vi "Save Archiving Parameters.vi"(5 "section":string, 7 "config ref in":T1, 8 "error in (no error)":errorcluster, 9 "2 LBCB Archiving Mode":bool, 10 "Log File Size (MBytes)":i64, 11 "Logging Directory":path) -> (0 "error out":errorcluster, 1 "config ref out":T1)   [LabVIEW 2013]
uses:
  <vilib>/Utility/config.llb/Config Data RefNum.ctl
  <vilib>/Utility/config.llb/Write Key (Path).vi
  <vilib>/Utility/config.llb/Write Key (Double).vi
  <vilib>/Utility/config.llb/Write Key (Boolean).vi
  <vilib>/Utility/config.llb/NI_LVConfig.lvlib
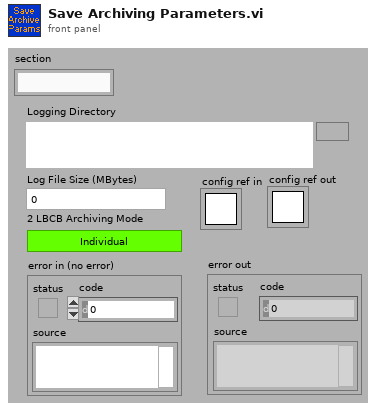
[diagram p1: front panel]
types:
  T1 = typedef "NI_LVConfig.lvlib/Config Data RefNum.ctl" = refnum<k1>
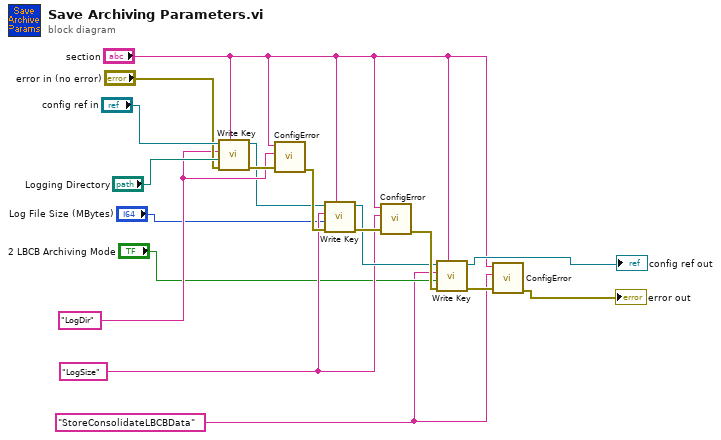
[diagram p0: block diagram]
diagram:
  w1 = "StoreConsolidateLBCBData" ("key")
  w4 = "LogSize" ("key")
  w14 = "LogDir" ("key")
  n1 = call-poly <vilib>:"Write Key.vi"("section"="section", "error in (no error)"="error in (no error)", "value"="Logging Directory", "key"=w14, "refnum"="config ref in") -> ("error out"=w15:errorcluster, "refnum out"=w8:T1)  [unwired: 4 in, 1 out]
  n2 = call "ConfigError.vi"("error in (no error)"=w15, "Key"=w14, "Section"="section") -> ("error out"=w11:errorcluster)  [unwired: 8 in]
  n3 = call-poly <vilib>:"Write Key.vi"("section"="section", "error in (no error)"=w11, "value"="Log File Size (MBytes)", "key"=w4, "refnum"=w8) -> ("error out"=w13:errorcluster, "refnum out"=w7:T1)  [unwired: 4 in, 1 out]
  n4 = call "ConfigError.vi"("error in (no error)"=w13, "Key"=w4, "Section"="section") -> ("error out"=w10:errorcluster)  [unwired: 8 in]
  n5 = call-poly <vilib>:"Write Key.vi"("section"="section", "error in (no error)"=w10, "value"="2 LBCB Archiving Mode", "key"=w1, "refnum"=w7) -> ("error out"=w12:errorcluster, "refnum out"=→"config ref out":T1)  [unwired: 4 in, 1 out]
  n6 = call "ConfigError.vi"("error in (no error)"=w12, "Key"=w1, "Section"="section") -> ("error out"=→"error out":errorcluster)  [unwired: 8 in]
